vi "DestroyPrivateEvents.vi"(8 "error in (no error)":errorcluster, 11 "MAUI":refnum<class "SMO.UI.MAUI.lvclass">) -> (0 "error out":errorcluster, 3 "MAUI out":refnum<class "SMO.UI.MAUI.lvclass">)   [LabVIEW 2019, in "SMO.UI.MAUI.lvclass"]
doc: "JKI State Machine Objects (SMO) 1.0.0.5\nJKI - JKI\nCopyright (c) 2016, JKI"
uses:
  SMO.UI.MAUI.lvclass
  <vilib>/JKI/JKI SMO/SMO.UI/SMO.UI.lvclass
panel:
  # "For instructions on how to use the JKI State Machine Objects, examples and video tutorials, visit:\nhttp://jki.net/state-machine-objects/\n\nJKI State Machine Objects™\nhttp://jki.net/state-machine-objects/\nCopyright (C) 2005-2015, JKI <info@jki.net>\nALL RIGHTS RESERVED"
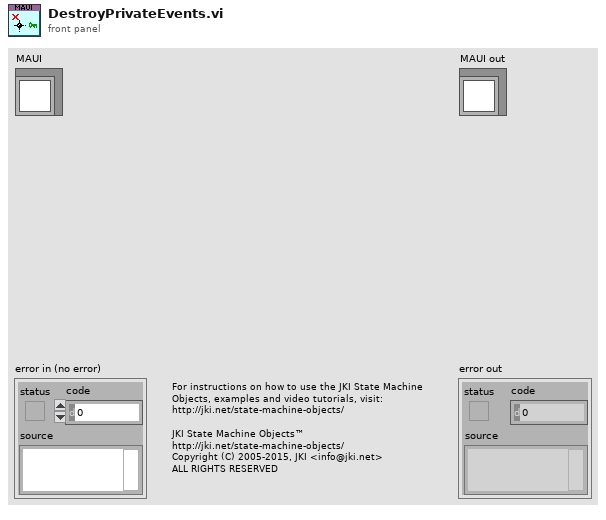
[diagram p1: front panel]
types:
  T1 = typedef "SMO.UI.MAUI.lvclass/PrivateEvents--Cluster.ctl" = cluster{"SetEmbedded":refnum<user-event>, "GetEmbedded":refnum<user-event>, "SetPanelData":refnum<user-event>, "GetPanelData":refnum<user-event>, "UpdatePanel":refnum<user-event>, "PopSubpanel":refnum<user-event>, "GetDefaultSubpanel":refnum<user-event>, "SetDefaultSubpanel":refnum<user-event>}
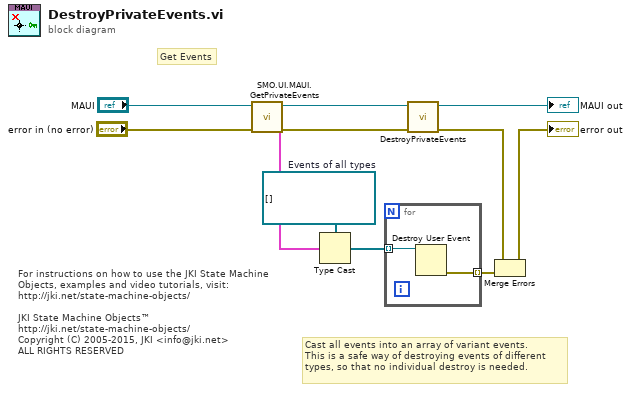
[diagram p0: block diagram]
diagram:
  w5 = refnum<user-event>[] []  # Events of all types
  # "Get Events"
  # "For instructions on how to use the JKI State Machine Objects, examples and video tutorials, visit:\nhttp://jki.net/state-machine-objects/\n\nJKI State Machine Objects™\nhttp://jki.net/state-machine-objects/\nCopyright (C) 2005-2015, JKI <info@jki.net>\nALL RIGHTS RESERVED"
  # "Cast all events into an array of variant events.\nThis is a safe way of destroying events of different\ntypes, so that no individual destroy is needed."
  n1 = call "SMO.UI.MAUI.GetPrivateEvents.vi"("error in (no error)"="error in (no error)", "MAUI"="MAUI") -> ("error out"=w8:errorcluster, "Private Events"=w1:T1, "MAUI out"=w3:refnum<class "SMO.UI.MAUI.lvclass">)  [unwired: 7 in]
  n2 = Type Cast(type=w5, x=w1) -> (*(type *) &x=w6:refnum<user-event>[])
  n3 = for {
    tunnel: w6 -> [w12] mode=indexing
    tunnel: [w13] -> w4 mode=indexing
    n4 = Destroy User Event(user event=w12) -> (error out=w13:errorcluster)  [unwired: 1 in]
  }
  n5 = call-parent "DestroyPrivateEvents.vi"("error in (no error)"=w8, "SMO.UI"=w3) -> ("error out"=w11:errorcluster, "SMO.UI out"=→"MAUI out":refnum<class "SMO.UI.MAUI.lvclass">)  [unwired: 8 in]
  n6 = Merge Errors(w11, w4) -> (→"error out":errorcluster)
